vi "Get Elapsed Time.vi"(7 "[x]":T1, 8 "error in (no error)":errorcluster, 11 "Serial Port in":refnum<visa-resource-name>) -> (0 "error out":errorcluster, 1 "Time string":string, 3 "Serial Port out":refnum<visa-resource-name>)   [LabVIEW 2020, in "Chemyx_Syringe_Pump_driver.lvlib"]
doc: "Returns the elapsed time of the current operation of the pump as a number of seconds and as a string formatted as X hr YY min ZZ sec."
uses:
  Chemyx_Syringe_Pump_driver.lvlib
  _private/Control/Control Mode.ctl
panel:
  out "Time (sec)":dbl
  # "Returns the elapsed time of the current operation of the pump as a number of seconds and as a string formatted as X hr YY min ZZ sec."
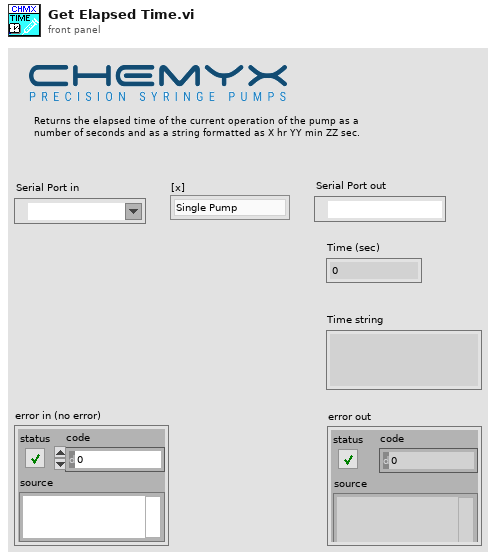
[diagram p1: front panel]
types:
  T1 = typedef "Chemyx_Syringe_Pump_driver.lvlib/Control Mode.ctl" = enum16{"Single Pump", "Pump Channel 1", "Pump Channel 2", "Cycle Mode"}
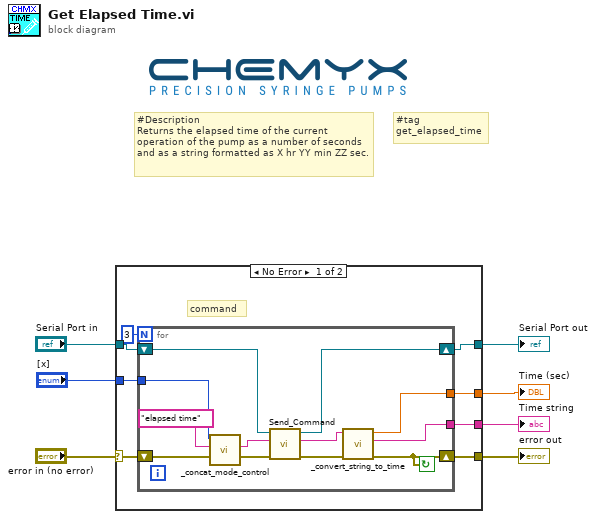
[diagram p0: block diagram]
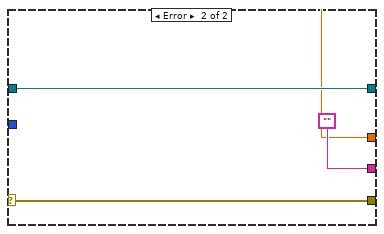
[diagram p2: hidden frame]
diagram:
  # "#tag\nget_elapsed_time"
  # "#Description\nReturns the elapsed time of the current operation of the pump as a number of seconds and as a string formatted as X hr YY min ZZ sec."
  n1 = case shown="No Error" "error in (no error)" {
    selector: "error in (no error)" -> [w14 w30]
    tunnel: "Serial Port in" -> [w15 w29]
    tunnel: [w10 "" ("read buffer")] -> w5
    tunnel: [w12 w30] -> w4
    tunnel: [w13 w29] -> w3
    tunnel: [w11 0.0] -> w2
    tunnel: "[x]" -> [w9 _]
    frame No Error {
      # "command"
      n2 = for {
        N: 3 -> [_]
        tunnel: [w21] -> w11
        tunnel: [w20] -> w10
        tunnel: w9 -> [w17]
        shift-right: [w23] -> w13
        shift-left: w15 -> [w26]
        shift-right: [w16] -> w12
        shift-left: w14 -> [w25]
        stop <- w16 continue-if-true
        n3 = call "_concat_mode_control.vi"("write buffer"="elapsed time", "[x]"=w17) -> ("write buffer out"=w18:string)  [unwired: 9 in]
        n4 = call "Send_Command.vi"("error in (no error)"=w25, "write buffer"=w18, "Serial Port in"=w26) -> ("error out"=w24:errorcluster, "Read buffer"=w22:string, "VISA Refnum out"=w23:refnum<visa-resource-name>)  [unwired: 6 in]
        n5 = call "_convert_string_to_time.vi"("error in (no error)"=w24, "Input string"=w22) -> ("error out"=w16:errorcluster, "Time String"=w20:string, "Time in seconds"=w21:dbl)  [unwired: 7 in]
      }
    }
    frame Error {
    }
  }
  "error out" <- w4
  "Serial Port out" <- w3
  "Time string" <- w5
  "Time (sec)" <- w2
